vi "Read GIF file.vi"(4 "image index":i32, 6 "bgcolor":u32(colorbox)=11776947, 8 "error in (no error)":errorcluster, 10 "String":string) -> (0 "error out":errorcluster, 2 "image data":T1)   [LabVIEW 2011]
doc: "Reads the selected image from a gif file and creates the data necessary to display the file in a picture control."
uses:
  <vilib>/picture/picture.llb/imagedata.ctl
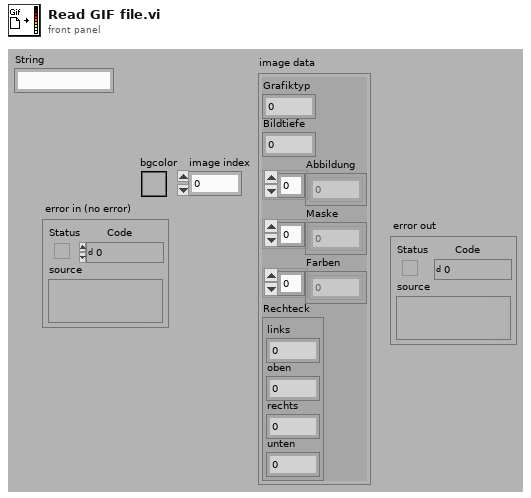
[diagram p1: front panel]
types:
  T1 = typedef "imagedata.ctl" = cluster{"image type":i32, "image depth":i32, "image":u8[], "mask":u8[], "colors":u32[], "Rectangle":cluster{"left":i16, "top":i16, "right":i16, "bottom":i16}}
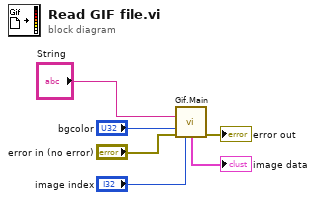
[diagram p0: block diagram]
diagram:
  n1 = call "Gif.Main.vi"("String"="String", "bgcolor"="bgcolor", "error in (no error)"="error in (no error)", "image index"="image index") -> ("image data"=→"image data":T1, "error out"=→"error out":errorcluster)  [unwired: 1 in, 9 out]
